vi "initialise.vi"(8 "error in (no error)":errorcluster, 11 "StageMG100204SutterMP285 in":refnum<class "StageMG100204SutterMP285.lvclass">=refnum) -> (0 "error out":errorcluster, 3 "StageMG100204SutterMP285 out":refnum<class "StageMG100204SutterMP285.lvclass">)   [LabVIEW 2010, in "StageMG100204SutterMP285.lvclass"]
doc: "The dynamic dispatch-version of this VI initalises the plug-in object by allocating and initalising any dynamic resources need."
uses:
  StageMG100204SutterMP285.lvclass
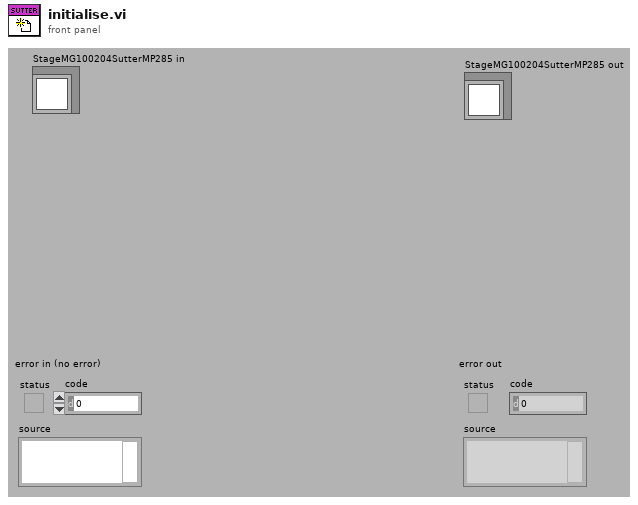
[diagram p1: front panel]
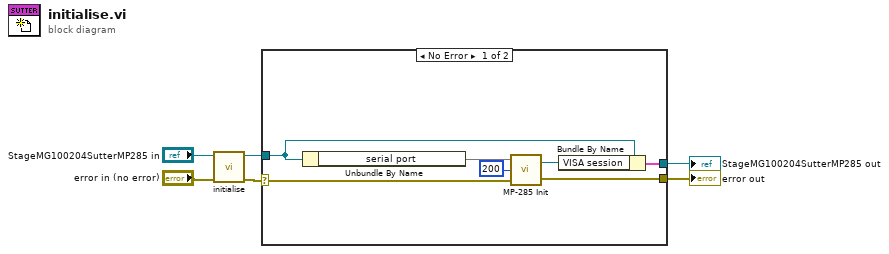
[diagram p0: block diagram]
diagram:
  n1 = call-parent "initialise.vi"("error in (no error)"="error in (no error)", "GenericPlugin in"="StageMG100204SutterMP285 in") -> ("error out"=w5:errorcluster, "GenericPlugin out"=w4:refnum<class "StageMG100204SutterMP285.lvclass">)  [unwired: 8 out]
  n2 = case shown="No Error" w5 {
    selector: w5 -> [w8 w14]
    tunnel: w4 -> [w11 w15]
    tunnel: [w10 w15] -> w2
    tunnel: [w13 w14] -> w3
    frame No Error {
      n3 = Unbundle By Name(w11) -> ("serial port"=w12)
      n4 = call "MP-285 Init.vi"("Input: Error Cluster"=w8, "Timeout (msec)"=u32 200, "Serial port # \n(COM1 - #1)!!!"=w12) -> ("error out"=w13:errorcluster, "reference out"=w9:refnum<visa-resource-name>)
      n5 = Bundle By Name(cluster=w11, "VISA session"=w9) -> (w10:cluster{})
    }
    frame Error {
    }
  }
  "error out" <- w3
  "StageMG100204SutterMP285 out" <- w2
